vi "ExpandItem__slk_tc.vi"(0 "tree control in":refnum<class "TreeControl.lvclass">, 5 "input tag (current tag)":string, 11 "error in (no error)":errorcluster) -> (4 "tree control out":refnum<class "TreeControl.lvclass">, 15 "error out":errorcluster)   [LabVIEW 2020, in "TreeControl.lvclass"]
doc: "Expands item by specified tag. If input tag is BLANK or unwired, it will use current tag. Ignore ENABLE if no selection."
uses:
  Library/TreeControl.lvclass
  Library/TreeControl.lvclass/TreeControl.ctl
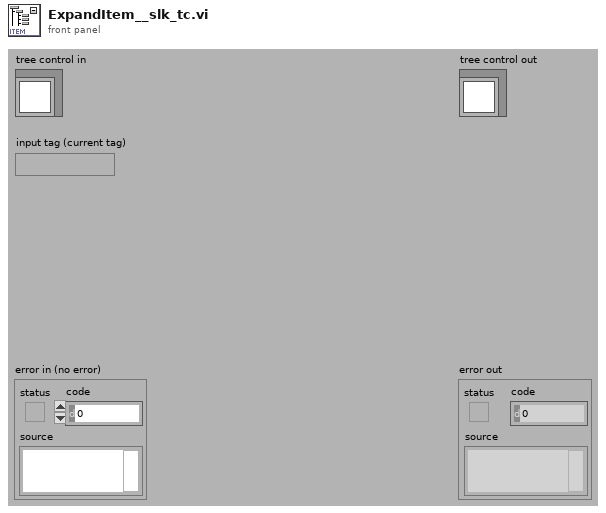
[diagram p1: front panel]
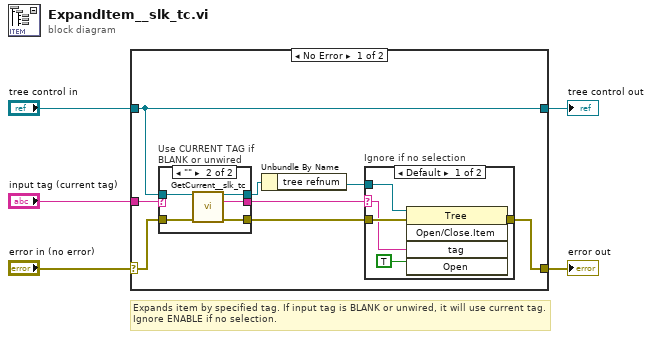
[diagram p0: block diagram]
diagram:
  # "Expands item by specified tag. If input tag is BLANK or unwired, it will use current tag. Ignore ENABLE if no selection."
  n1 = case shown="No Error" "error in (no error)" {
    selector: "error in (no error)" -> [w7 w29]
    tunnel: [w6 w29] -> w4
    tunnel: [w13 w28] -> w2
    tunnel: "tree control in" -> [w13 w28]
    tunnel: "input tag (current tag)" -> [w12 _]
    frame No Error {
      n2 = case "Use CURRENT TAG if BLANK or unwired" shown="\"\"" w12 {
        selector: w12 -> [w22 _]
        tunnel: [w22 w27] -> w11
        tunnel: w13 -> [w20 w26]
        tunnel: w7 -> [w21 w25]
        tunnel: [w21 w24] -> w10
        tunnel: [w20 w23] -> w9
        frame Default {
        }
        frame "" {
          n3 = call "GetCurrent__slk_tc.vi"("tree control in"=w26, "error in (no error)"=w25) -> ("tree control out"=w23:refnum<class "TreeControl.lvclass">, "current tag"=w27:string, "error out"=w24:errorcluster)  [unwired: 1 in, 10 out]
        }
      }
      n4 = Unbundle By Name(w9) -> ("tree refnum"=w8:refnum<vi>)
      n5 = case "Ignore if no selection" shown="Default" w11 {
        selector: w11 -> [w15 _]
        tunnel: w10 -> [w18 w19]
        tunnel: w8 -> [w17 _]
        tunnel: [w16 w19] -> w6
        frame Default {
          n6 = invoke class="Tree" method="Open/Close.Item"(reference=w17, error in=w18, "tag"=w15, "Open"=TRUE ("Open?")) -> (error out=w16:errorcluster)  [unwired: 1 in, 4 out]
        }
        frame "" {
        }
      }
    }
    frame Error {
    }
  }
  "error out" <- w4
  "tree control out" <- w2
